vi "CSM - Filter Duplicate Messages By Name.vi"(6 "Whole Messages in Check?(T)":bool=TRUE, 11 "States":string="abc >> 1\nabc  >> 2\ndef\nabc >> 3\n121212\nabc >> 4") -> (3 "States out":string="abc >> 4\r\ndef\r\n121212")   [LabVIEW 2020, in "Communicable State Machine.lvlib"]
uses:
  Communicable State Machine.lvlib
  Match Regular Expression.xnode
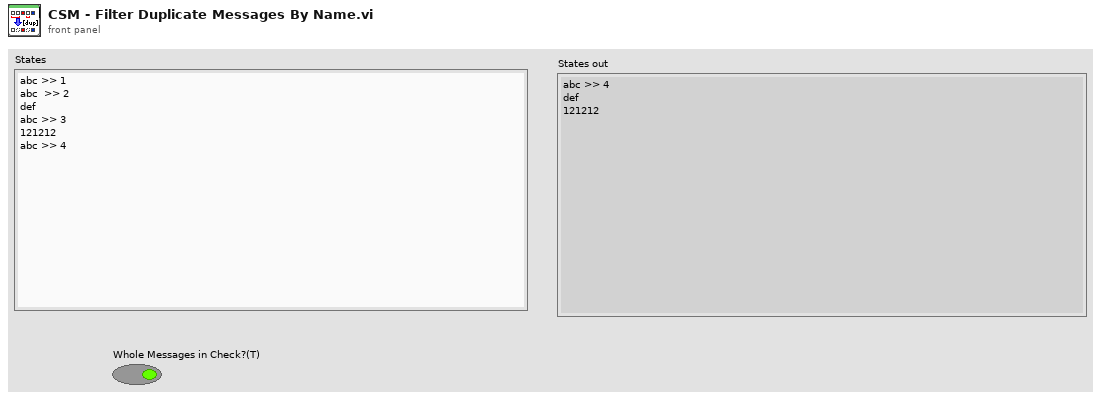
[diagram p1: front panel]
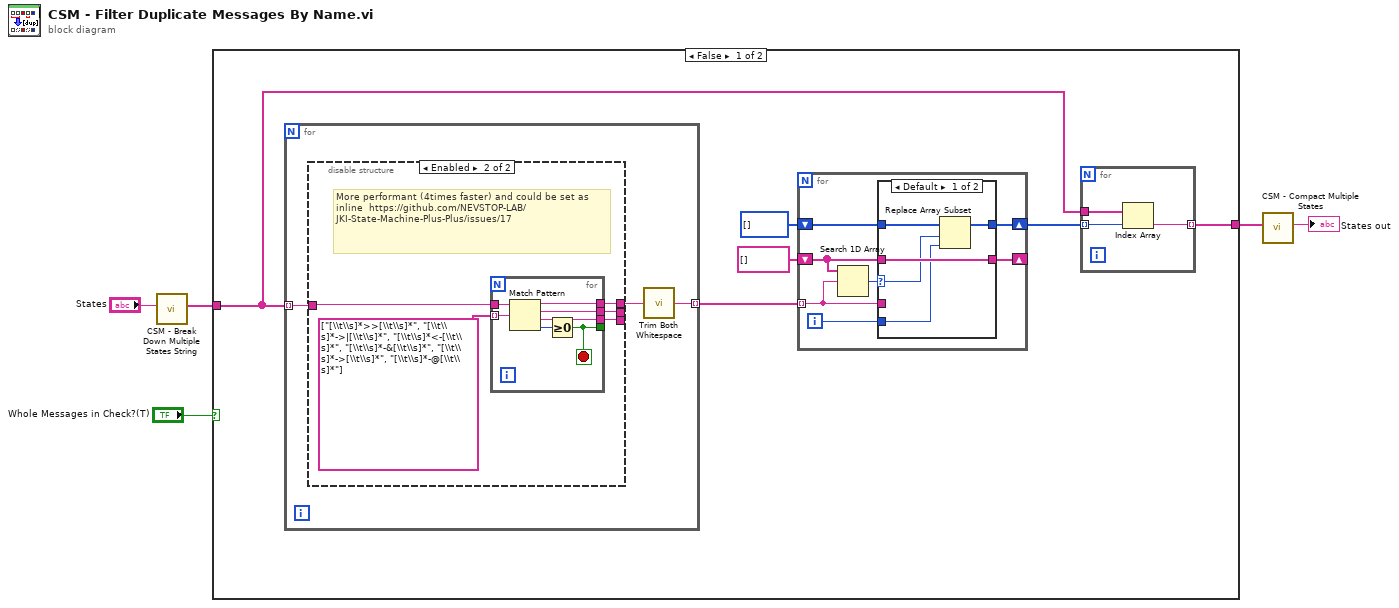
[diagram p0: block diagram]
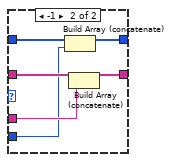
[diagram p2: hidden frame]
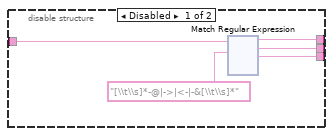
[diagram p3: hidden frame]
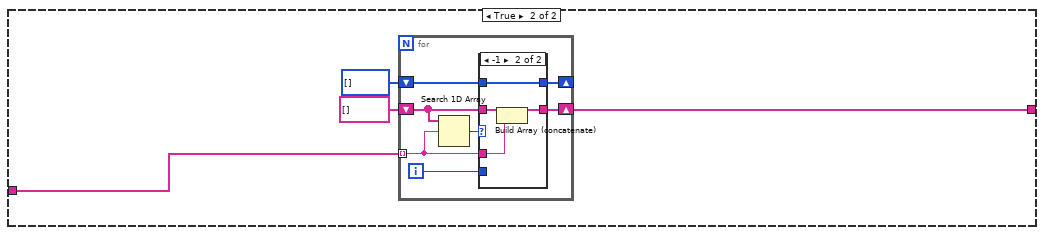
[diagram p4: hidden frame]
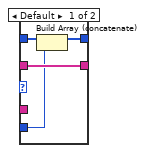
[diagram p5: hidden frame]
diagram:
  n1 = call "CSM - Break Down Multiple States String.vi"("States"="States") -> ("Multiple States"=w4:string[])  [unwired: 10 in]
  n2 = case shown="False" "Whole Messages in Check?(T)" {
    tunnel: w4 -> [w10 w168]
    tunnel: [w9 w167] -> w3
    frame False {
      n3 = for {
        tunnel: w10 -> [w35] mode=indexing
        tunnel: [w33] -> w11 mode=indexing
        n4 = disable-structure shown="Enabled" {
          disable-tunnel: [w39 w157] -> w34
          disable-tunnel: [w38 w156] -> _
          disable-tunnel: [w37 w155] -> _
          disable-tunnel: w35 -> [w36 w159]
          frame Disabled {
            n5 = xnode "Match Regular Expression"("input string"=w36, "regular expression"="[\\t\\s]*-@|->|<-|-&[\\t\\s]*") -> ("before match"=w39:string, "whole match"=w38:string, "after match"=w37:string)  [unwired: 4 in, 2 out]
          }
          frame Enabled {
            # "More performant (4times faster) and could be set as inline  https://github.com/NEVSTOP-LAB/JKI-State-Machine-Plus-Plus/issues/17"
            n6 = for {
              tunnel: w159 -> [w166]
              tunnel: string[] ["[\\t\\s]*>>[\\t\\s]*", "[\\t\\s]*->|[\\t\\s]*", "[\\t\\s]*<-[\\t\\s]*", "[\\t\\s]*-&[\\t\\s]*", "[\\t\\s]*->[\\t\\s]*", "[\\t\\s]*-@[\\t\\s]*"] -> [w165] mode=indexing
              tunnel: [w163] -> _
              tunnel: [w162] -> w157
              tunnel: [w161] -> w156
              tunnel: [w160] -> w155
              stop <- w163 stop-if-true
              n7 = Match Pattern(string=w166, regular expression=w165) -> (before substring=w162:string, match substring=w161:string, after substring=w160:string, offset past match=w164:i32)  [unwired: 1 in]
              n8 = Greater Or Equal To 0?(x=w164) -> (x >= 0?=w163:bool)
            }
          }
        }
        n9 = call "Trim Both Whitespace.vi"("string"=w34) -> ("trimmed string"=w33:string)  [unwired: 1 in]
      }
      n10 = for {
        tunnel: w11 -> [w20] mode=indexing
        shift-right: [w19] -> _
        shift-left: string[] [] -> [w18]
        shift-right: [w16] -> w6
        shift-left: i32[] [] -> [w15]
        i -> [w17]
        n11 = Search 1D Array(1D array=w18, element=w20) -> (index of element=w21:i32)  [unwired: 1 in]
        n12 = case shown="Default" w21 {
          selector: w21 -> [w23 _]
          tunnel: w20 -> [_ w32]
          tunnel: [w26 w30] -> w19
          tunnel: w18 -> [w26 w31]
          tunnel: w17 -> [w22 w27]
          tunnel: [w24 w28] -> w16
          tunnel: w15 -> [w25 w29]
          frame Default {
            n13 = Replace Array Subset(array=w25, new element=w22, index=w23) -> (w24:i32[])
          }
          frame -1 {
            n14 = Build Array (concatenate)(w29, w27) -> (w28:i32[])
            n15 = Build Array (concatenate)(w31, w32) -> (w30:string[])
          }
        }
      }
      n16 = for {
        tunnel: w6 -> [w14] mode=indexing
        tunnel: w10 -> [w13]
        tunnel: [w12] -> w9 mode=indexing
        n17 = Index Array(array=w13, index=w14) -> (element=w12:string)
      }
    }
    frame True {
      n18 = for {
        tunnel: w168 -> [w176] mode=indexing
        shift-right: [w175] -> w167
        shift-left: string[] [] -> [w174]
        shift-right: [w172] -> _
        shift-left: i32[] [] -> [w171]
        i -> [w173]
        n19 = Search 1D Array(1D array=w174, element=w176) -> (index of element=w177:i32)  [unwired: 1 in]
        n20 = case shown="-1" w177 {
          tunnel: w176 -> [_ w185]
          tunnel: [w181 w183] -> w175
          tunnel: w174 -> [w181 w184]
          tunnel: w173 -> [w178 _]
          tunnel: [w179 w182] -> w172
          tunnel: w171 -> [w180 w182]
          frame Default {
            n21 = Build Array (concatenate)(w180, w178) -> (w179:i32[])
          }
          frame -1 {
            n22 = Build Array (concatenate)(w184, w185) -> (w183:string[])
          }
        }
      }
    }
  }
  n23 = call "CSM - Compact Multiple States.vi"("Multiple States"=w3) -> ("States"=→"States out":string)  [unwired: 9 in]
